vi "verify process.vi"() -> ()   [LabVIEW 2014]
panel:
  out "NeedRestart?":bool
  in  "data out 2":string
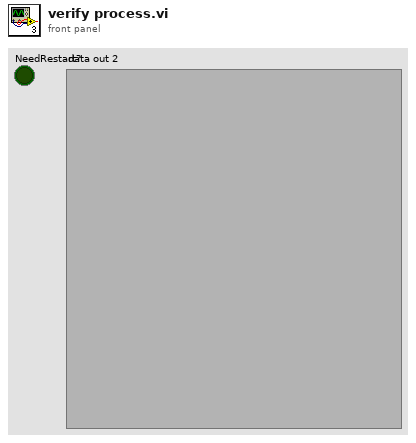
[diagram p1: front panel]
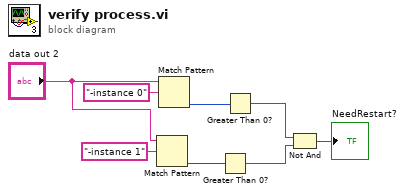
[diagram p0: block diagram]
diagram:
  n1 = Match Pattern(string="data out 2", regular expression="-instance 1") -> (offset past match=w6:i32)  [unwired: 1 in, 3 out]
  n2 = Match Pattern(string="data out 2", regular expression="-instance 0") -> (offset past match=w5:i32)  [unwired: 1 in, 3 out]
  n3 = Greater Than 0?(x=w6) -> (x > 0?=w2:bool)
  n4 = Greater Than 0?(x=w5) -> (x > 0?=w3:bool)
  n5 = Not And(1:w2, 2:w3) -> (0:→"NeedRestart?":bool)
